vi "TEST_NAME.vi"(1 "call chain":string[](array[string])) -> (0 "String":string)   [LabVIEW 2013]
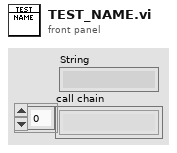
[diagram p1: front panel]
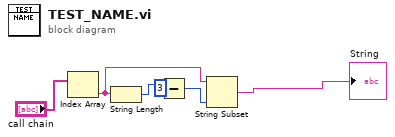
[diagram p0: block diagram]
diagram:
  n1 = Index Array(array="call chain") -> (element=w4:string)  [unwired: 1 in]
  n2 = String Length(string=w4) -> (length=w2:i32)
  n3 = Subtract(x=w2, y=3 ("length (rest)")) -> (x-y=w5:i32)
  n4 = String Subset(string=w4, length (rest)=w5) -> (substring=→"String":string)  [unwired: 1 in]
